vi "detectPotentialFieldBlock.vi"(8 "error in (no error)":errorcluster, 10 "v_tang/v_norm resultant":dbl[](array[numeric]), 11 "Robot in":refnum<class "Robot.lvclass">) -> (0 "error out":errorcluster, 2 "potentialFieldBlockedRobot":bool, 3 "Robot out":refnum<class "Robot.lvclass">)   [LabVIEW 2023, in "Robot.lvclass"]
uses:
  Robot.lvclass
  Robot.lvclass/Robot.ctl
  <vilib>/Analysis/_algsub.llb/Real Vector Norm.vi
  <vilib>/Analysis/baseanly.llb/Real Dot Product.vi
  Read v_tang.vi
  Read v_norm.vi
  <vilib>/Analysis/NI_AALPro.lvlib
  <vilib>/Analysis/NI_AALBase.lvlib
  Utilities_class/Utilities.lvclass
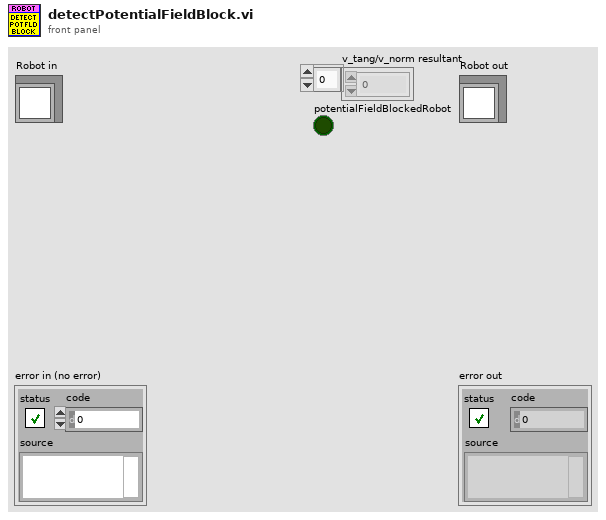
[diagram p1: front panel]
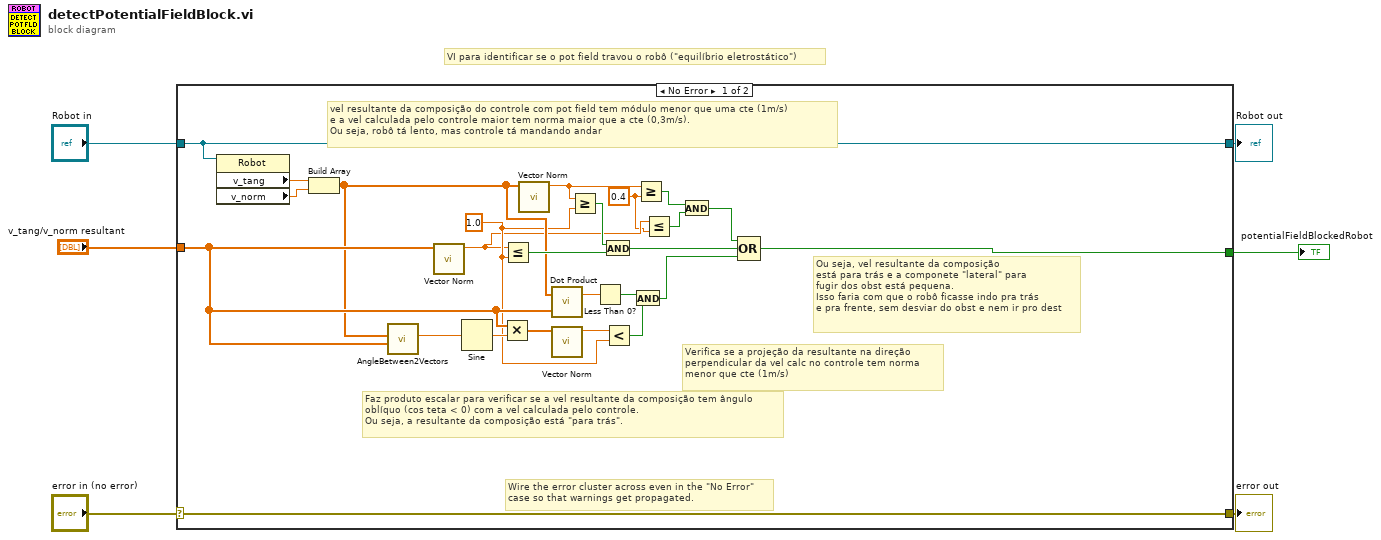
[diagram p0: block diagram]
diagram:
  # "VI para identificar se o pot field travou o robô (\"equilíbrio eletrostático\")"
  n1 = case shown="No Error" "error in (no error)" {
    selector: "error in (no error)" -> [w31 w33]
    tunnel: [w31 w33] -> w5
    tunnel: [w29 w32] -> w3
    tunnel: "Robot in" -> [w29 w32]
    tunnel: "v_tang/v_norm resultant" -> [w19 _]
    tunnel: [w14 _] -> w1
    frame No Error {
      w9 = 0.4 ("y")
      w11 = 1.0 ("y")
      # "Ou seja, vel resultante da composição\nestá para trás e a componete \"lateral\" para\nfugir dos obst está pequena.\nIsso faria com que o robô ficasse indo pra trás\ne pra frente, sem desviar do obst e nem ir pro dest"
      # "Verifica se a projeção da resultante na direção\nperpendicular da vel calc no controle tem norma\nmenor que cte (1m/s)"
      # "Faz produto escalar para verificar se a vel resultante da composição tem ângulo\noblíquo (cos teta < 0) com a vel calculada pelo controle.\nOu seja, a resultante da composição está \"para trás\"."
      # "vel resultante da composição do controle com pot field tem módulo menor que uma cte (1m/s)\ne a vel calculada pelo controle maior tem norma maior que a cte (0,3m/s).\nOu seja, robô tá lento, mas controle tá mandando andar"
      # "Wire the error cluster across even in the \"No Error\"\ncase so that warnings get propagated."
      n2 = property class="Robot"(reference=w29) -> ("v_tang"=w28:dbl, "v_norm"=w27:dbl)  [unwired: 1 in, 2 out]
      n3 = Build Array(w28, w27) -> (w18:dbl[])
      n4 = call "AngleBetween2Vectors.vi"("Array 1"=w19, "Array 2"=w18) -> ("angleInRadians(default)"=w21:dbl)  [unwired: 6 in, 3 out]
      n5 = call-poly <vilib>:"Vector Norm.vi"("Input Vector"=w19) -> ("norm"=w10:dbl)  [unwired: 9 in, 1 out]
      n6 = Sine(x=w21) -> (sin(x)=w20:dbl)
      n7 = Multiply(x=w19, y=w20) -> (x*y=w17:dbl[])
      n8 = Less Or Equal?(x=w10, y=w11) -> (x <= y?=w30:bool)
      n9 = call-poly <vilib>:"Vector Norm.vi"("Input Vector"=w18) -> ("norm"=w13:dbl)  [unwired: 9 in, 1 out]
      n10 = call-poly <vilib>:"Dot Product.vi"("Y Vector"=w19, "X Vector"=w18) -> ("X * Y"=w24:dbl)  [unwired: 1 out]
      n11 = call-poly <vilib>:"Vector Norm.vi"("Input Vector"=w17) -> ("norm"=w16:dbl)  [unwired: 9 in, 1 out]
      n12 = Greater Or Equal?(x=w13, y=w11) -> (x >= y?=w26:bool)
      n13 = Less Than 0?(x=w24) -> (x < 0?=w23:bool)
      n14 = And(x=w26, y=w30) -> (x .and. y?=w25:bool)
      n15 = Less?(x=w16, y=w11) -> (x < y?=w15:bool)
      n16 = And(x=w23, y=w15) -> (x .and. y?=w22:bool)
      n17 = Greater Or Equal?(x=w13, y=w9) -> (x >= y?=w12:bool)
      n18 = Less Or Equal?(x=w10, y=w9) -> (x <= y?=w8:bool)
      n19 = And(x=w12, y=w8) -> (x .and. y?=w7:bool)
      n20 = Compound Arithmetic op=OR(w7, w25, w22) -> (w14:bool)
    }
    frame Error {
    }
  }
  "error out" <- w5
  "Robot out" <- w3
  "potentialFieldBlockedRobot" <- w1
